vi "Find overlattice using co-incident search 2015-1-8.vi"(6 "Minimal Angle from GB plane":dbl, 7 "Minimal thickness of the grain (A)":dbl=0.05, 8 "Co-incidence Tolerance":dbl=0.05, 9 "Number of integers to search":i32=50, 10 "Mutual Viewing Angle":dbl[](array[numeric])=[0.0, 1.0, 0.0], 11 "Grain Boundary Macro Definition":T1={"Grain 1 Orientation"=[1.0, 0.0, 0.0], "Grain 2 Orientation"=[0.707, 0.707, 0.0], "Twist Angle (Deg)"=0.0}) -> (1 "Perpendicular to GB Plane, Lattice c":dbl[](array[numeric]), 2 "GB Plane 2, Lattice b":dbl[](array[numeric]), 3 "GB Plane 1, Lattice a":dbl[](array[numeric]))   [LabVIEW 2010]
panel:
  out "Angle (Degrees)":dbl
  out "deleted portion":dbl[](array[numeric])
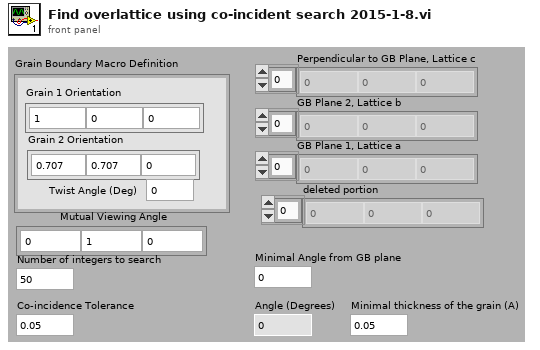
[diagram p1: front panel]
types:
  T1 = cluster{"Grain 1 Orientation":dbl[], "Grain 2 Orientation":dbl[], "Twist Angle (Deg)":dbl}
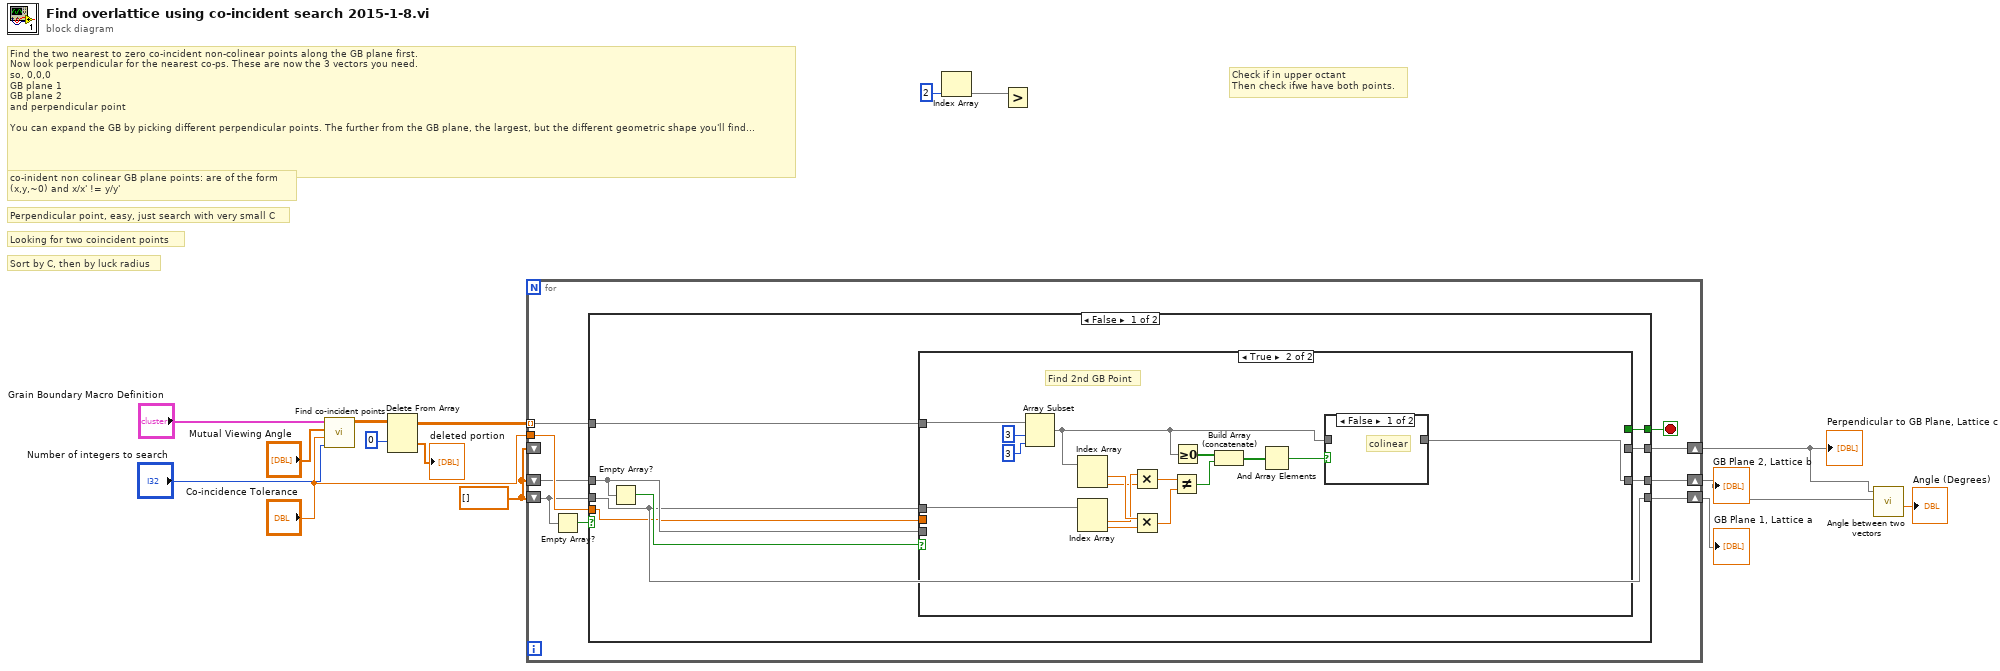
[diagram p0: block diagram]
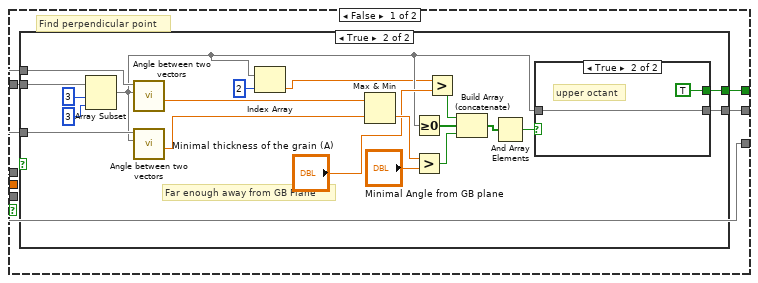
[diagram p2: hidden frame]
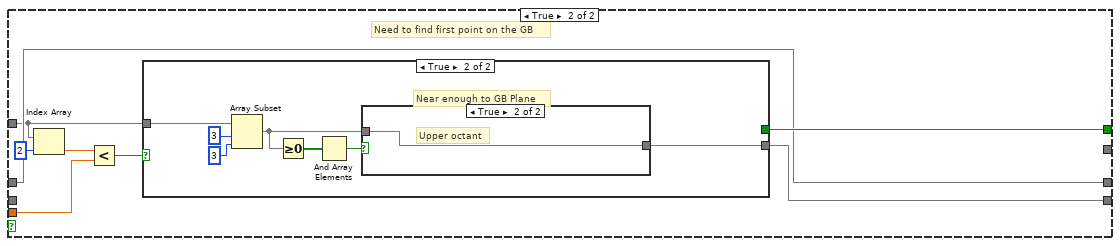
[diagram p6: hidden frame]
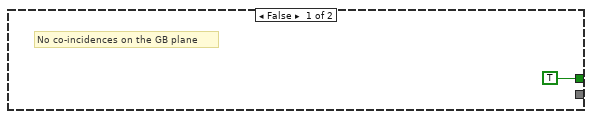
[diagram p7: hidden frame]
diagram:
  w12 = dbl[] []
  # "Check if in upper octant\nThen check ifwe have both points."
  # "Looking for two coincident points"
  # "Sort by C, then by luck radius"
  # "Perpendicular point, easy, just search with very small C"
  # "co-inident non colinear GB plane points: are of the form\n(x,y,~0) and x/x' != y/y'"
  # "Find the two nearest to zero co-incident non-colinear points along the GB plane first.\nNow look perpendicular for the nearest co-ps. These are now the 3 vectors you need. \nso, 0,0,0\nGB plane 1\nGB plane 2\nand perpendicular point\n\nYou can expand the GB by picking different perpendicular points. The further from the GB plane, the largest, but the different geometric shape you'll find..."
  n1 = call "Find co-incident points.vi"("Half of the number of integers to search"="Number of integers to search", "Co-incidence Tolerance"="Co-incidence Tolerance", "Mutual Viewing Angle"="Mutual Viewing Angle", "Grain Boundary Macro Definition"="Grain Boundary Macro Definition") -> ("Coincident points"=w15:dbl[][])  [unwired: 7 in]
  n2 = Delete From Array(array=w15, index (row)=0) -> (deleted portion=→"deleted portion":dbl[], array with subset deleted=w13:dbl[][])  [unwired: 2 in]
  n3 = for {
    tunnel: w13 -> [w17] mode=indexing
    shift-right: [w23] -> w8
    shift-left: w12 -> [w20]
    tunnel: "Co-incidence Tolerance" -> [w24]
    shift-right: [w19] -> w5
    shift-left: w12 -> [w21]
    shift-right: [w18] -> w6
    shift-left: w12 -> [_]
    stop <- w22 stop-if-true
    n4 = Empty Array?(array=w20) -> (empty?=w25:bool)
    n5 = case shown="False" w25 {
      tunnel: w17 -> [w31 w80]
      tunnel: w24 -> [w28 w85]
      tunnel: [w30 w83] -> w23
      tunnel: [w26 w82] -> w22
      tunnel: w21 -> [w32 w81]
      tunnel: w20 -> [w30 _]
      tunnel: [w29 w81] -> w19
      tunnel: [w27 _] -> w18
      frame False {
        n6 = Empty Array?(array=w32) -> (empty?=w33:bool)
        n7 = case shown="True" w33 {
          tunnel: w32 -> [w34 _]
          tunnel: w31 -> [w38 w67]
          tunnel: w30 -> [w35 w71]
          tunnel: [w34 w70] -> w29
          tunnel: w28 -> [_ _]
          tunnel: [w37 _] -> w27
          tunnel: [w36 _] -> w26
          frame False {
            # "Find perpendicular point"
            n8 = case shown="True" w39 {
              tunnel: w38 -> [_ w56]
              tunnel: [_ w54] -> w37
              tunnel: [_ w57] -> w36
              tunnel: w35 -> [_ w53]
              tunnel: w34 -> [_ w52]
              frame False {
                # "Not far enough away from the GB Plane"
              }
              frame True {
                # "Far enough away from GB Plane"
                n9 = Array Subset(array=w56, index=3, length=3) -> (w42:dbl[])
                n10 = call "Angle between two vectors.vi"("Vector 2"=w42, "Vector 1"=w53) -> ("Angle (Degrees)"=w50:dbl)  [unwired: 7 in, 2 out]
                n11 = call "Angle between two vectors.vi"("Vector 2"=w42, "Vector 1"=w52) -> ("Angle (Degrees)"=w51:dbl)  [unwired: 7 in, 2 out]
                n12 = Index Array(array=w42, index=2) -> (element=w40:dbl)
                n13 = Max & Min(x=w50, y=w51) -> (min(x,y)=w49:dbl)  [unwired: 1 out]
                n14 = Greater Or Equal To 0?(x=w42) -> (x >= 0?=w46:bool[])
                n15 = Greater?(x=w49, y="Minimal Angle from GB plane") -> (0:w47:bool)
                n16 = Greater?(x=w40, y="Minimal thickness of the grain (A)") -> (0:w44:bool)
                n17 = Build Array (concatenate)(w44, w46, w47) -> (w45:bool[])
                n18 = And Array Elements(Boolean array=w45) -> (logical AND=w55:bool)
                n19 = case shown="True" w55 {
                  tunnel: [_ TRUE] -> w57
                  tunnel: [_ w60] -> w54
                  tunnel: w42 -> [_ w60]
                  frame False {
                    # "elsewhere"
                  }
                  frame True {
                    # "upper octant"
                  }
                }
              }
            }
          }
          frame True {
            # "Find 2nd GB Point"
            n20 = Array Subset(array=w67, index=3, length=3) -> (w62:dbl[])
            n21 = Index Array(array=w62) -> (element #1=w77:dbl, element #2=w74:dbl)  [unwired: 2 in]
            n22 = Index Array(array=w71) -> (element #1=w75:dbl, element #2=w76:dbl)  [unwired: 2 in]
            n23 = Multiply(x=w75, y=w74) -> (x*y=w73:dbl)
            n24 = Multiply(x=w77, y=w76) -> (x*y=w72:dbl)
            n25 = Not Equal?(x=w73, y=w72) -> (x != y?=w65:bool)
            n26 = Greater Or Equal To 0?(x=w62) -> (x >= 0?=w66:bool[])
            n27 = Build Array (concatenate)(w66, w65) -> (w64:bool[])
            n28 = And Array Elements(Boolean array=w64) -> (logical AND=w63:bool)
            n29 = case shown="False" w63 {
              tunnel: [_ w78] -> w70
              tunnel: w62 -> [_ w78]
              frame False {
                # "colinear"
              }
              frame True {
              }
            }
          }
        }
      }
      frame True {
        # "Need to find first point on the GB"
        n30 = Index Array(array=w80, index=2) -> (element=w86:dbl)
        n31 = Less?(x=w86, y=w85) -> (x < y?=w84:bool)
        n32 = case shown="True" w84 {
          tunnel: w80 -> [_ w92]
          tunnel: [_ w88] -> w83
          tunnel: [TRUE _] -> w82
          frame False {
            # "No co-incidences on the GB plane"
          }
          frame True {
            # "Near enough to GB Plane"
            n33 = Array Subset(array=w92, index=3, length=3) -> (w89:dbl[])
            n34 = Greater Or Equal To 0?(x=w89) -> (x >= 0?=w91:bool[])
            n35 = And Array Elements(Boolean array=w91) -> (logical AND=w90:bool)
            n36 = case shown="True" w90 {
              tunnel: [_ w95] -> w88
              tunnel: w89 -> [_ w95]
              frame False {
                # "Elsewhere"
              }
              frame True {
                # "Upper octant"
              }
            }
          }
        }
      }
    }
  }
  "Perpendicular to GB Plane, Lattice c" <- w6
  "GB Plane 2, Lattice b" <- w5
  "GB Plane 1, Lattice a" <- w8
  n37 = Index Array(index=2) -> (element=w1)  [unwired: 1 in]
  n38 = Greater?(x=w1) -> (y=w2:dbl)  [unwired: 1 out]
  n39 = call "Angle between two vectors.vi"("Vector 2"=w5, "Vector 1"=w6) -> ("Angle (Degrees)"=→"Angle (Degrees)":dbl)  [unwired: 7 in, 2 out]
